vi "Configure Timebase Mode.vi"(8 "error in (no error)":errorcluster, 10 "Timebase Mode (0: YT)":u16(ring) items=["YT", "XY", "Roll"], 11 "VISA resource name":refnum<visa-resource-name>) -> (0 "error out":errorcluster, 3 "VISA resource name out":refnum<visa-resource-name>)   [LabVIEW 2015, in "RIGOL DS1000 Series.lvlib"]
doc: "Configures timebase mode of the oscilloscope."
uses:
  RIGOL DS1000 Series.lvlib
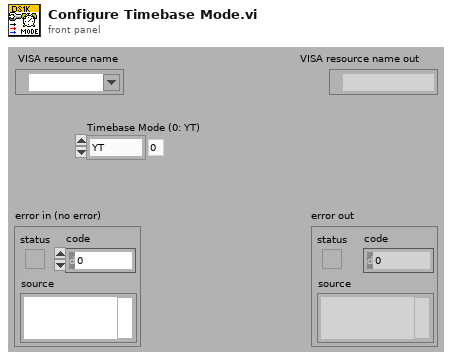
[diagram p1: front panel]
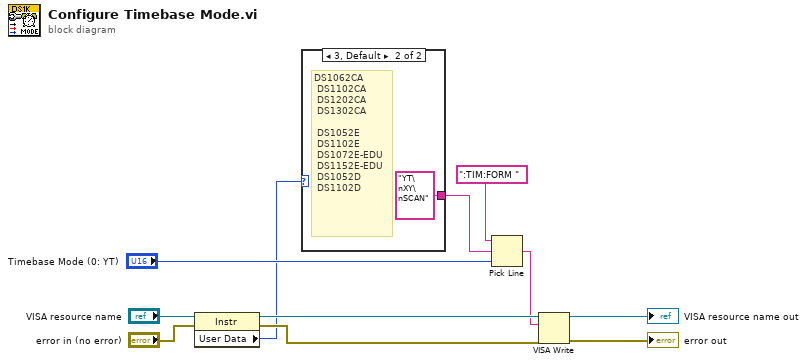
[diagram p0: block diagram]
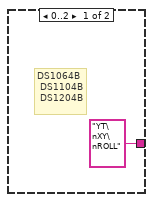
[diagram p2: hidden frame]
diagram:
  n1 = property class="Instr"(reference="VISA resource name", error in="error in (no error)") -> (reference out=w4:refnum<visa-resource-name>, error out=w3:errorcluster, "User Data"=w1:u32)
  n2 = case shown="3, Default" w1 {
    tunnel: ["YT\nXY\nROLL" ("multi-line string") "YT\nXY\nSCAN" ("multi-line string")] -> w10
    frame 0..2 {
      # "DS1064B\n DS1104B\n DS1204B"
    }
    frame 3, Default {
      # "DS1062CA\n DS1102CA\n DS1202CA\n DS1302CA\n\n DS1052E\n DS1102E\n DS1072E-EDU\n DS1152E-EDU\n DS1052D\n DS1102D"
    }
  }
  n3 = Pick Line(string ("")=":TIM:FORM ", multi-line string=w10, line index="Timebase Mode (0: YT)") -> (output string=w2:string)
  n4 = VISA Write(VISA resource name=w4, write buffer=w2, error in (no error)=w3) -> (VISA resource name out=→"VISA resource name out":refnum<visa-resource-name>, error out=→"error out":errorcluster)  [unwired: 1 out]
